vi "CreateSelfReference.vi"(8 "error in (no error)":errorcluster, 11 "OPM.ThorlabsPM400":refnum<class "OPM.ThorlabsPM400.lvclass">) -> (0 "error out":errorcluster, 3 "OPM.ThorlabsPM400 out":refnum<class "OPM.ThorlabsPM400.lvclass">)   [LabVIEW 2017, in "OPM.ThorlabsPM400.lvclass"]
doc: "JKI State Machine Objects (SMO) 1.0.0.5\nJKI - JKI\nCopyright (c) 2016, JKI"
uses:
  OPM.ThorlabsPM400.lvclass
  OPM.ThorlabsPM400.lvclass/OPM.ThorlabsPM400.ctl
  <vilib>/JKI/JKI SMO/SMO/SMO.lvclass
panel:
  # "For instructions on how to use the JKI State Machine Objects, examples and video tutorials, visit:\nhttp://jki.net/state-machine-objects/\n\nJKI State Machine Objects™\nhttp://jki.net/state-machine-objects/\nCopyright (C) 2005-2015, JKI <info@jki.net>\nALL RIGHTS RESERVED"
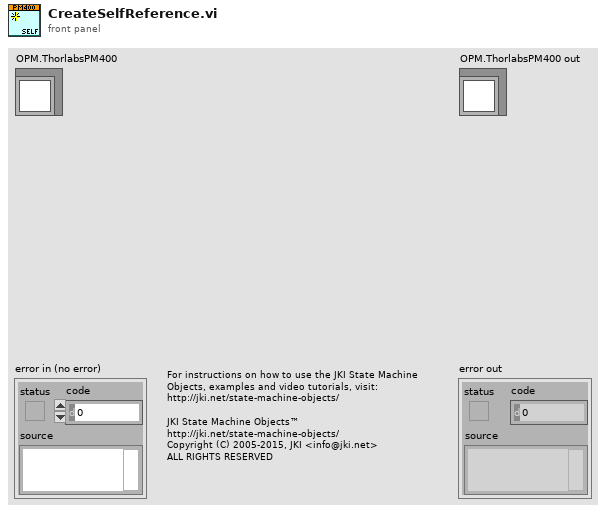
[diagram p1: front panel]
types:
  T1 = typedef "OPM.ThorlabsPM400.lvclass/PrivateData--Ref.ctl" = refnum<data-value>
  T2 = typedef "OPM.ThorlabsPM400.lvclass/PrivateData--Cluster.ctl" = cluster{"Resource":T3}
  T3 = typedef "OPM.ThorlabsPM400.lvclass/Resource--Cluster.ctl" = cluster{"Instrument handle":refnum<visa-resource-name>}
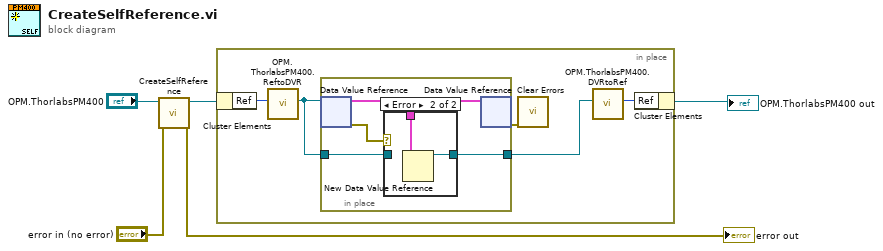
[diagram p0: block diagram]
diagram:
  n1 = call-parent "CreateSelfReference.vi"("error in (no error)"="error in (no error)", "SMO"="OPM.ThorlabsPM400") -> ("error out"=→"error out":errorcluster, "SMO out"=w4:refnum<class "OPM.ThorlabsPM400.lvclass">)  [unwired: 8 in]
  n2 = in-place {
    n3 = in-place-cluster #1(w4) -> ("Ref"=w10:u32)
    n4 = call "OPM.ThorlabsPM400.ReftoDVR.vi"("Ref"=w10) -> ("Ref"=w9:T1)  [unwired: 10 in]
    n5 = in-place {
      in-place-border: [w14] -> w7
      in-place-border: w9 -> [w11]
      n6 = in-place-dvr #2(w9) -> (w13:T2, w12:errorcluster)
      n7 = case shown="Error" w12 {
        tunnel: [w15 w17] -> w14
        tunnel: w13 -> [_ w16]
        tunnel: w11 -> [w15 _]
        frame No Error {
        }
        frame Error {
          n8 = New Data Value Reference(data value=w16) -> (data value reference=w17:refnum<data-value>)  [unwired: 1 in, 1 out]
        }
      }
      n9 = in-place-dvr #2(w13) -> (w6:errorcluster)  [unwired: 1 out]
    }
    n10 = call <vilib>:"Clear Errors.vi"("error in (no error)"=w6) -> ()  [unwired: 5 in, 2 out]
    n11 = call "OPM.ThorlabsPM400.DVRtoRef.vi"("Ref"=w7) -> ("Ref"=w8:u32)  [unwired: 10 in]
    n12 = in-place-cluster #1("Ref"=w8) -> (→"OPM.ThorlabsPM400 out":refnum<class "OPM.ThorlabsPM400.lvclass">)
  }
